vi "Scale Replay DBL Data to DAC Codes.vi"(11 "replay data":dbl[](array[numeric])) -> (3 "DAC data":i16[](array[numeric]))   [LabVIEW 2013, in "Engine Simulation Toolkit System Explorer.lvlib"]
uses:
  Engine Simulation Toolkit System Explorer.lvlib
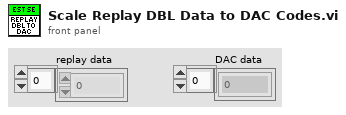
[diagram p1: front panel]
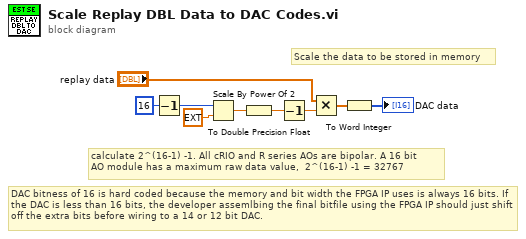
[diagram p0: block diagram]
diagram:
  # "DAC bitness of 16 is hard coded because the memory and bit width the FPGA IP uses is always 16 bits. If the DAC is less than 16 bits, the developer assemlbing the final bitfile using the FPGA IP should just shift off the extra bits before wiring to a 14 or 12 bit DAC."
  # "calculate 2^(16-1) -1. All cRIO and R series AOs are bipolar. A 16 bit\nAO module has a maximum raw data value,  2^(16-1) -1 = 32767"
  # "Scale the data to be stored in memory"
  n1 = Decrement(x=u8 16 ("DAC bit resolution")) -> (x-1=w4:u8)
  n2 = Scale By Power Of 2(n=w4, x=ext 1.0) -> (x*2^n=w3:ext)
  n3 = To Double Precision Float(number=w3) -> (double precision float=w1:dbl)
  n4 = Decrement(x=w1) -> (x-1=w2:dbl)
  n5 = Multiply(x="replay data", y=w2) -> (x*y=w7:dbl[])
  n6 = To Word Integer(number=w7) -> (16bit integer=→"DAC data":i16[])
